vi "Lian_Lab02_I2.vi"() -> ()   [LabVIEW 2020]
uses:
  <vilib>/measure/NI_MABase.lvlib
panel:
  out "Iteration Count":i32
  out "Waveform Graph":waveform(dbl)(graph)
  in  "Stop":bool
  out "Waveform Chart":waveform(dbl)(graph)
  in  "frequency":dbl=10.0 format="%0.2p"
  in  "amplitude":dbl=1.0 format="%0.2p"
  in  "phase":dbl format="%.2p"
  in  "sampling info":cluster{"Fs":dbl, "#s":dbl}={"Fs"=1000.0, "#s"=1000.0} {"Fs" format="%.2p"}
  in  "offset":dbl format="%0.2p"
  # "Waveform Chart While Loop with Active User Control"
  # "Note: Panel objects are locked. Unlock to access additional features."
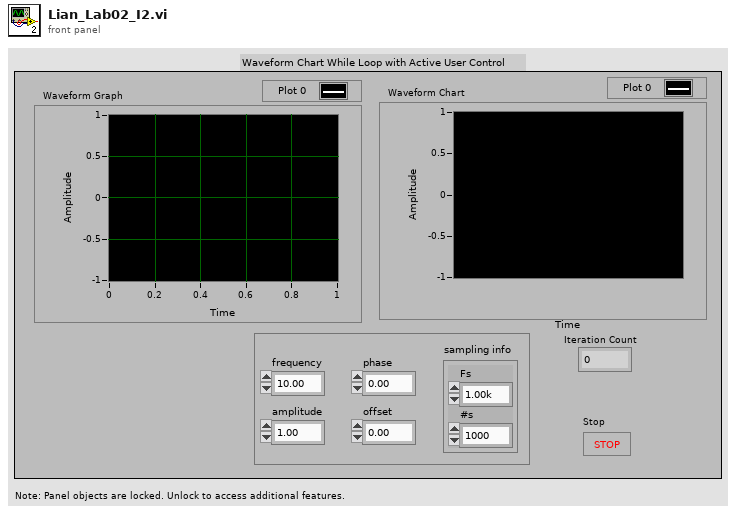
[diagram p1: front panel]
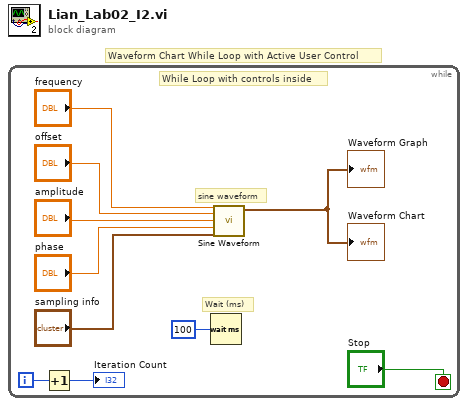
[diagram p0: block diagram]
diagram:
  # "Waveform Chart While Loop with Active User Control"
  n1 = while {
    i -> [w2]
    stop <- "Stop" stop-if-true
    # "While Loop with controls inside"
    # "Wait (ms)"
    # "sine waveform"
    n2 = Increment(x=w2) -> (x+1=→"Iteration Count":i32)
    n3 = Wait (ms)(milliseconds to wait=u32 100) -> ()  [unwired: 1 out]
    n4 = call <vilib>:"Sine Waveform.vi"("offset"="offset", "sampling info"="sampling info", "phase"="phase", "amplitude"="amplitude", "frequency"="frequency") -> ("signal out"=→"Waveform Graph" →"Waveform Chart":waveform(dbl))  [unwired: 5 in, 1 out]
  }
